vi "Exercitiu 10+11.vi"() -> ()   [LabVIEW 2023]
panel:
  out "Rezultat":string
  in  "b":string
  out "Numar caractere text a":dbl
  in  "a":string
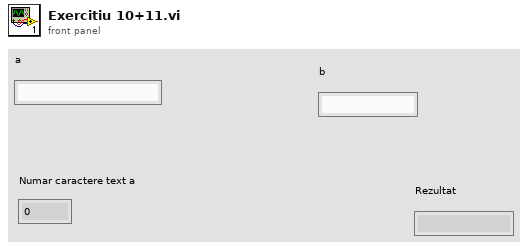
[diagram p1: front panel]
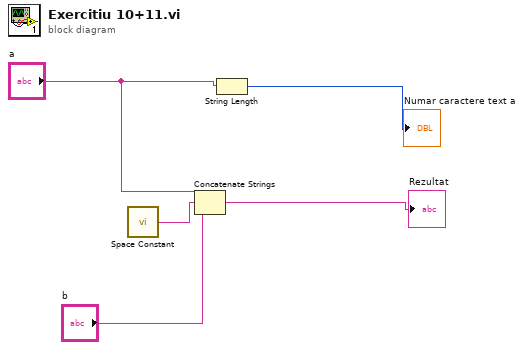
[diagram p0: block diagram]
diagram:
  n1 = call <vilib>:"Space Constant.vi"() -> ("String"=w3:string)
  n2 = Concatenate Strings("a", w3, "b") -> (→"Rezultat":string)
  n3 = String Length(string="a") -> (length=→"Numar caractere text a":i32)
